vi "0xFA_Cmd_programreset_(SubVI).vi"(11 "String in":string) -> (3 "String out":string)   [LabVIEW 2017, in "LV_Unicorn.lvlib"]
uses:
  LV_Unicorn.lvlib
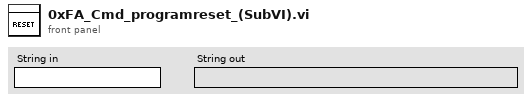
[diagram p1: front panel]
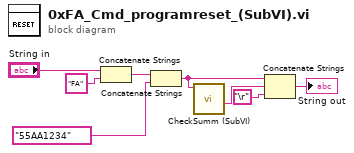
[diagram p0: block diagram]
diagram:
  n1 = Concatenate Strings("String in", "FA" ("string")) -> (w6:string)
  n2 = Concatenate Strings(w6, "55AA1234" ("string")) -> (w3:string)
  n3 = call "CheckSumm (SubVI).vi"("Input String"=w3) -> ("CheckSumm"=w2:string)  [unwired: 7 in, 3 out]
  n4 = Concatenate Strings(w3, w2, "\r") -> (→"String out":string)
